vi "ProcExec.vi"(0 "ProcessName":string="cmd", 1 "Stop Button Ref":refnum<vi>, 3 "StreamWrite String Ref":refnum<vi>, 5 "arguments":string, 7 "Timeout (ms)":i32=-1, 9 "Output File Path":path, 12 "StreamOut String Ref":refnum<vi>, 14 "StreamErr String Ref":refnum<vi>) -> (15 "error out":errorcluster)   [LabVIEW 2017]
doc: "Open process specified in <B>ProcessName</B> in interactive or non interactive mode.\n\n<B>arguments</B>: arguments passed to process to excute.\n<B>StreamWrite String Ref</B>: if this control is not empty the process will be opened in interactive mode. Limit to single option shall be enabled into string associated to ref passed in for working correctly.\n<B>Timeout (ms)</B>: this control is valid only in non interactive mode. Wait process exit for given time. If time is -1 wait indefinitely.\n<B>Output File Path</B>: output process stream will be saved into passed file. If this control is empty or invalid no file will be generated."
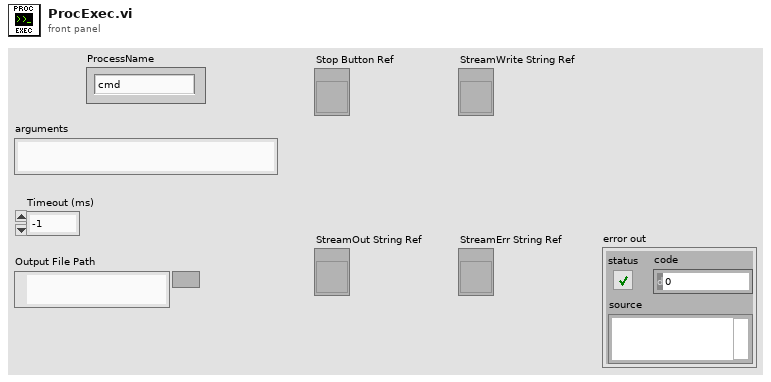
[diagram p1: front panel]
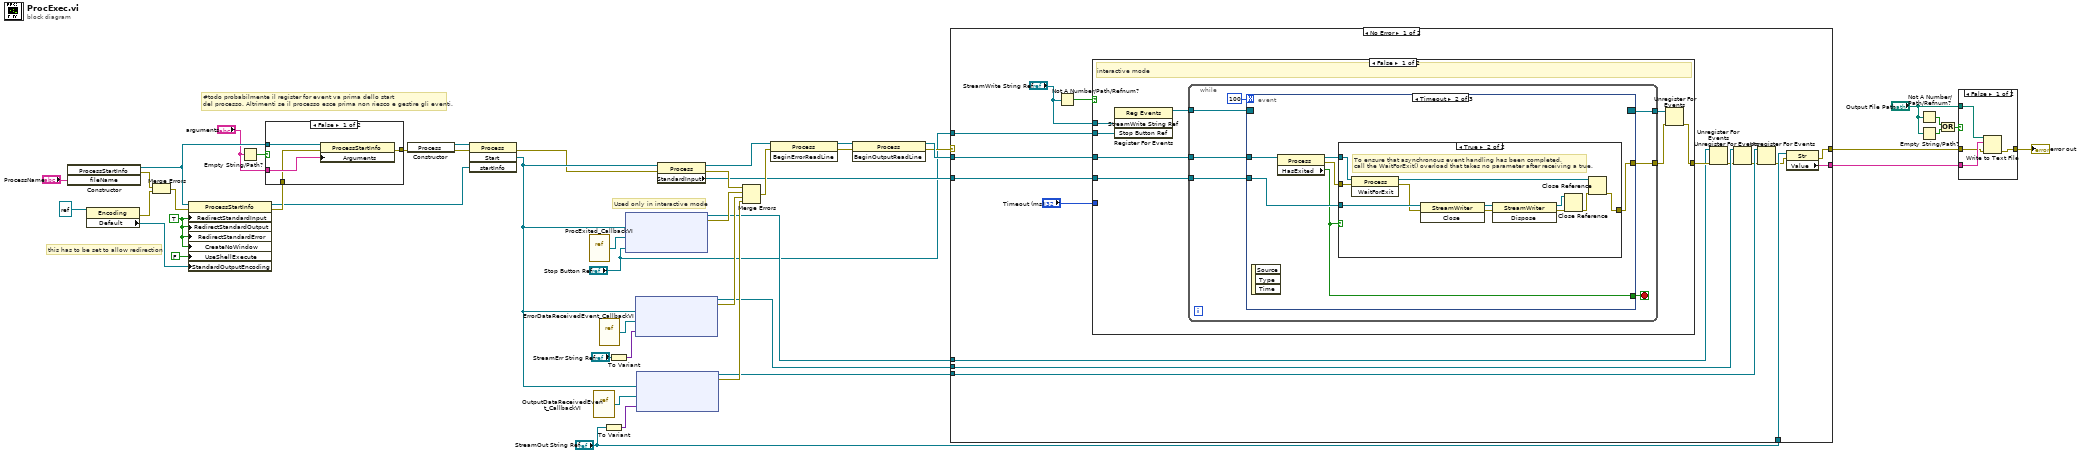
[diagram p0: block diagram]
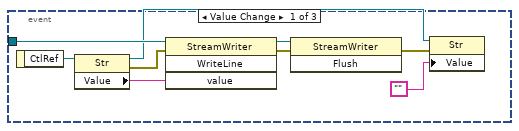
[diagram p3: hidden frame]
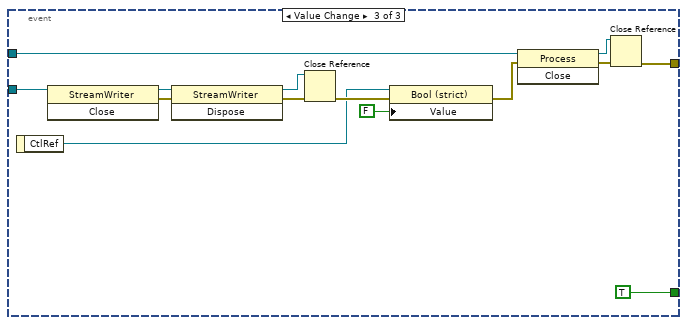
[diagram p5: hidden frame]
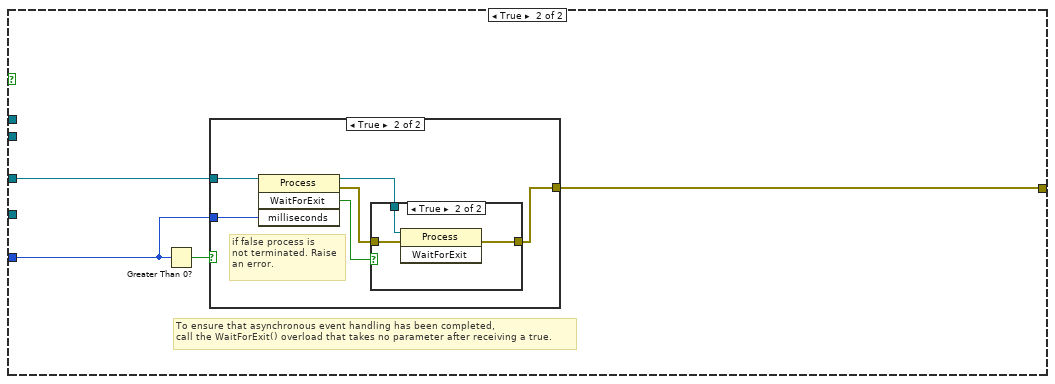
[diagram p6: hidden frame]
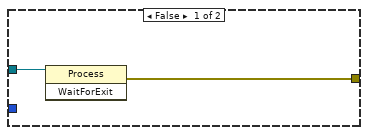
[diagram p7: hidden frame]
diagram:
  w10 = TRUE ("RedirectStandardInput")
  # "#todo probabilmente il register for event va prima dello start\ndel processo. Altrimenti se il processo esce prima non riesco e gestire gli eventi."
  # "Used only in interactive mode"
  # "this has to be set to allow redirection"
  n1 = constructor class="ProcessStartInfo"("fileName"="ProcessName") -> (reference out=w25:refnum<k24>, error out=w13:errorcluster)  [unwired: 3 in, 2 out]
  n2 = property class="Encoding"(reference=refnum<k24> refnum ("StandardOutputEncoding")) -> (error out=w12:errorcluster, "Default"=w29:refnum<k24>)  [unwired: 1 in, 1 out]
  n3 = Merge Errors(w13, w12) -> (w11:errorcluster)
  n4 = property class="ProcessStartInfo"(reference=w25, error in=w11, "RedirectStandardInput"=w10, "RedirectStandardOutput"=w10, "RedirectStandardError"=w10, "CreateNoWindow"=w10, "UseShellExecute"=FALSE, "StandardOutputEncoding"=w29) -> (reference out=w17:refnum<k24>, error out=w26:errorcluster)
  n5 = Empty String/Path?(string/path="arguments") -> (empty?=w23:bool)
  n6 = case shown="False" w23 {
    tunnel: "arguments" -> [w51 _]
    tunnel: w25 -> [w50 _]
    tunnel: w26 -> [w49 w52]
    tunnel: [w48 w52] -> w28
    frame False {
      n7 = property class="ProcessStartInfo"(reference=w50, error in=w49, "Arguments"=w51) -> (error out=w48:errorcluster)  [unwired: 1 out]
    }
    frame True {
    }
  }
  n8 = constructor class="Process"(error in=w28) -> (reference out=w15:refnum<k24>, error out=w27:errorcluster)  [unwired: 2 in, 1 out]
  n9 = invoke class="Process" method="Start"(reference=w15, error in=w27, "startInfo"=w17) -> (error out=w22:errorcluster, "Start"=w37:refnum<k24>)  [unwired: 1 in, 2 out]
  n10 = vi-ref "ProcExited_CallbackVI.vi"() -> ("vi reference"=w21:refnum<vi>)
  n11 = vi-ref "OutputDataReceivedEvent_CallbackVI.vi"() -> ("vi reference"=w38:refnum<vi>)
  n12 = vi-ref "ErrorDataReceivedEvent_CallbackVI.vi"() -> ("vi reference"=w34:refnum<vi>)
  n13 = To Variant(anything="StreamOut String Ref") -> (Variant=w39:variant)
  n14 = To Variant(anything="StreamErr String Ref") -> (Variant=w36:variant)
  n15 = node(w37, w21, "Stop Button Ref") -> (w20:refnum<k27>, w31:errorcluster)  [unwired: 2 in]
  n16 = node(w37, w34, w36) -> (w7:refnum<k27>, w40:errorcluster)  [unwired: 2 in]
  n17 = node(w37, w38, w39) -> (w6:refnum<k27>, w41:errorcluster)  [unwired: 2 in]
  n18 = property class="Process"(reference=w37, error in=w22) -> (reference out=w42:refnum<k24>, error out=w30:errorcluster, "StandardInput"=w16:refnum<k24>)
  n19 = Merge Errors(w30, w31, w40, w41) -> (w46:errorcluster)
  n20 = invoke class="Process" method="BeginErrorReadLine"(reference=w42, error in=w46) -> (reference out=w44:refnum<k24>, error out=w45:errorcluster)  [unwired: 1 in, 1 out]
  n21 = invoke class="Process" method="BeginOutputReadLine"(reference=w44, error in=w45) -> (reference out=w43:refnum<k24>, error out=w9:errorcluster)  [unwired: 1 in, 1 out]
  n22 = case shown="No Error" w9 {
    selector: w9 -> [_ w141]
    tunnel: w16 -> [w68 _]
    tunnel: w20 -> [w63 _]
    tunnel: w43 -> [w53 _]
    tunnel: [w65 _] -> w47
    tunnel: "StreamOut String Ref" -> [w66 _]
    tunnel: "Stop Button Ref" -> [w67 _]
    tunnel: w7 -> [w62 _]
    tunnel: w6 -> [w61 _]
    tunnel: [w57 w141] -> w5
    frame No Error {
      n23 = Not A Number/Path/Refnum?(number/path/refnum="StreamWrite String Ref") -> (NaN/Path/Refnum?=w55:bool)
      n24 = case shown="False" w55 {
        tunnel: w68 -> [w76 _]
        tunnel: w53 -> [w75 w128]
        tunnel: w67 -> [w73 _]
        tunnel: "StreamWrite String Ref" -> [w72 _]
        tunnel: "Timeout (ms)" -> [_ w126]
        tunnel: [w69 w125] -> w64
        frame False {
          # "interactive mode"
          n25 = register-events(w72, w73) -> (reference out=w74:refnum<event-registration>)  [unwired: 2 in, 1 out]
          n26 = while {
            tunnel: w76 -> [w83]
            tunnel: w75 -> [w81]
            tunnel: w74 -> [w80]
            tunnel: [w79] -> w70
            tunnel: [w78] -> w71
            stop <- w82 stop-if-true
            n27 = event shown="[1] Timeout" {
              selector: w80 -> [_ _ _]
              dyn-events: [_ _ _] -> w78
              timeout: 100 -> [_ _ _]
              tunnel: w83 -> [w92 w97 w122]
              tunnel: [_ w96 TRUE] -> w82
              tunnel: w81 -> [_ w98 w123]
              tunnel: [_ w95 w111] -> w79
              event Value Change {
                n28 = event-data() -> ("CtlRef"=w87:refnum<vi>)  [unwired: 1 in]
                n29 = property on="Property Node" class="Str"(reference=w87) -> (reference out=w85:refnum<vi>, error out=w88:errorcluster, "Value"=w89:string)  [unwired: 1 in]
                n30 = invoke class="StreamWriter" method="WriteLine"(reference=w92, error in=w88, "value"=w89) -> (reference out=w91:refnum<k24>, error out=w90:errorcluster)  [unwired: 1 in, 2 out]
                n31 = invoke class="StreamWriter" method="Flush"(reference=w91, error in=w90) -> (error out=w86:errorcluster)  [unwired: 1 in, 2 out]
                n32 = property on="Property Node" class="Str"(reference=w85, error in=w86, "Value"="") -> ()  [unwired: 2 out]
              }
              event Timeout {
                n33 = event-data() -> ()  [unwired: 1 in, 3 out]
                n34 = property class="Process"(reference=w98) -> (reference out=w93:refnum<k24>, error out=w94:errorcluster, "HasExited"=w96:bool)  [unwired: 1 in]
                n35 = case shown="True" w96 {
                  tunnel: w97 -> [_ w106]
                  tunnel: w94 -> [w99 w104]
                  tunnel: [w99 w100] -> w95
                  tunnel: w93 -> [_ w105]
                  frame False {
                  }
                  frame True {
                    # "To ensure that asynchronous event handling has been completed,\ncall the WaitForExit() overload that takes no parameter after receiving a true."
                    n36 = invoke class="Process" method="WaitForExit"(reference=w105, error in=w104) -> (reference out=w102:refnum<k24>, error out=w103:errorcluster)  [unwired: 1 in, 1 out]
                    n37 = invoke class="StreamWriter" method="Close"(reference=w106, error in=w103) -> (reference out=w110:refnum<k24>, error out=w109:errorcluster)  [unwired: 1 in, 1 out]
                    n38 = invoke class="StreamWriter" method="Dispose"(reference=w110, error in=w109) -> (reference out=w107:refnum<k24>, error out=w108:errorcluster)  [unwired: 1 in, 1 out]
                    n39 = Close Reference(reference=w107, error in (no error)=w108) -> (error out=w101:errorcluster)
                    n40 = Close Reference(reference=w102, error in (no error)=w101) -> (error out=w100:errorcluster)
                  }
                }
              }
              event Value Change {
                n41 = event-data() -> ("CtlRef"=w113:refnum<vi>)  [unwired: 1 in]
                n42 = invoke class="StreamWriter" method="Close"(reference=w122) -> (reference out=w121:refnum<k24>, error out=w120:errorcluster)  [unwired: 2 in, 1 out]
                n43 = invoke class="StreamWriter" method="Dispose"(reference=w121, error in=w120) -> (reference out=w116:refnum<k24>, error out=w117:errorcluster)  [unwired: 1 in, 1 out]
                n44 = Close Reference(reference=w116, error in (no error)=w117) -> (error out=w114:errorcluster)
                n45 = property on="Property Node" class="Bool (strict)"(reference=w113, error in=w114, "Value"=FALSE ("Stop Button")) -> (error out=w112:errorcluster)  [unwired: 1 out]
                n46 = invoke class="Process" method="Close"(reference=w123, error in=w112) -> (reference out=w118:refnum<k24>, error out=w119:errorcluster)  [unwired: 1 in, 1 out]
                n47 = Close Reference(reference=w118, error in (no error)=w119) -> (error out=w111:errorcluster)
              }
            }
          }
          n48 = Unregister For Events(event registration refnum=w71, error in=w70) -> (error out=w69:errorcluster)
        }
        frame True {
          # "To ensure that asynchronous event handling has been completed,\ncall the WaitForExit() overload that takes no parameter after receiving a true."
          n49 = Greater Than 0?(x=w126) -> (x > 0?=w127:bool)
          n50 = case shown="True" w127 {
            tunnel: w128 -> [w130 w136]
            tunnel: w126 -> [_ w135]
            tunnel: [w129 w131] -> w125
            frame False {
              n51 = invoke class="Process" method="WaitForExit"(reference=w130) -> (error out=w129:errorcluster)  [unwired: 2 in, 2 out]
            }
            frame True {
              # "if false process is\nnot terminated. Raise\nan error."
              n52 = invoke class="Process" method="WaitForExit"(reference=w136, "milliseconds"=w135) -> (reference out=w133:refnum<k24>, error out=w132:errorcluster, "WaitForExit"=w134:bool)  [unwired: 2 in, 1 out]
              n53 = case shown="True" w134 {
                tunnel: w133 -> [_ w140]
                tunnel: w132 -> [w137 w139]
                tunnel: [w137 w138] -> w131
                frame False {
                }
                frame True {
                  n54 = invoke class="Process" method="WaitForExit"(reference=w140, error in=w139) -> (error out=w138:errorcluster)  [unwired: 1 in, 2 out]
                }
              }
            }
          }
        }
      }
      n55 = Unregister For Events(event registration refnum=w63, error in=w64) -> (error out=w60:errorcluster)
      n56 = Unregister For Events(event registration refnum=w62, error in=w60) -> (error out=w59:errorcluster)
      n57 = Unregister For Events(event registration refnum=w61, error in=w59) -> (error out=w58:errorcluster)
      n58 = property on="Property Node" class="Str"(reference=w66, error in=w58) -> (error out=w57:errorcluster, "Value"=w65:string)  [unwired: 1 out]
    }
    frame Error {
    }
  }
  n59 = Not A Number/Path/Refnum?(number/path/refnum="Output File Path") -> (NaN/Path/Refnum?=w2:bool)
  n60 = Empty String/Path?(string/path="Output File Path") -> (empty?=w3:bool)
  n61 = Or(x=w2, y=w3) -> (x .or. y?=w1:bool)
  n62 = case shown="False" w1 {
    tunnel: w47 -> [w145 _]
    tunnel: [w144 w146] -> w32
    tunnel: "Output File Path" -> [w143 _]
    tunnel: w5 -> [w142 w146]
    frame False {
      n63 = Write to Text File(file (use dialog)=w143, text=w145, error in=w142) -> (error out=w144:errorcluster)  [unwired: 1 in, 2 out]
    }
    frame True {
    }
  }
  "error out" <- w32
